vi "CThread Get VI Depends.vi"(4 "Counted Refs":string[](array[string]), 9 "Owning VI":refnum<vi>) -> (3 "Array":refnum<vi>[](array[refnum]))   [LabVIEW 2012, in "CThread.lvlib"]
uses:
  CThread.lvlib
  <vilib>/Utility/traverseref.llb/TRef TravTarget.ctl
  <vilib>/Utility/traverseref.llb/VI Scripting - Traverse.lvlib
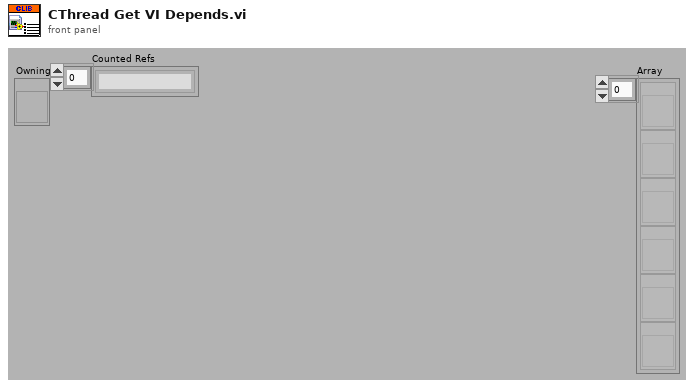
[diagram p1: front panel]
types:
  T1 = typedef "TRef TravTarget.ctl" = enum16{"FP", "BD", "Other"}
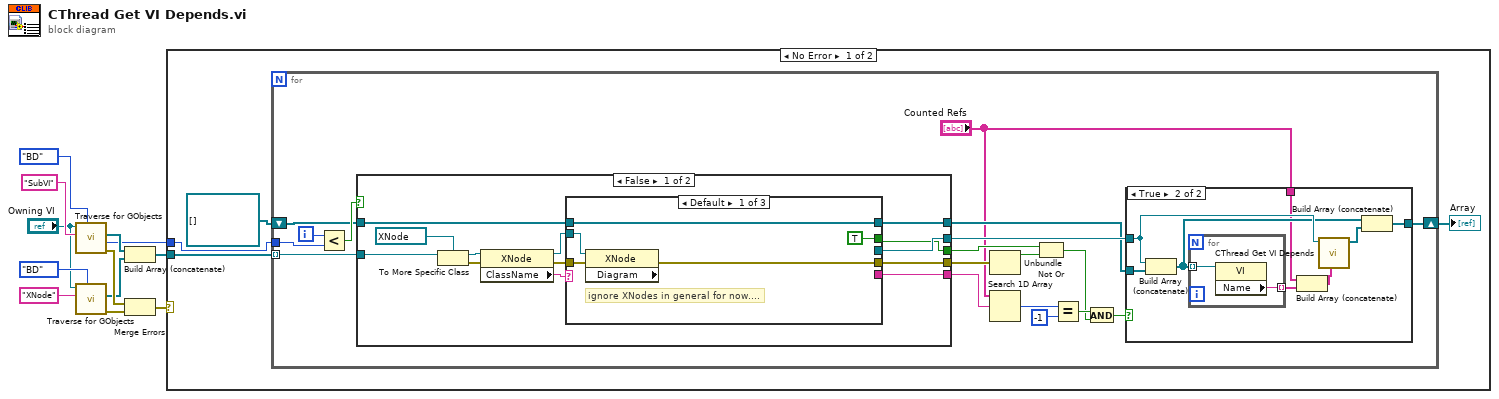
[diagram p0: block diagram]
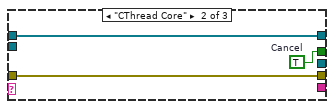
[diagram p2: hidden frame]
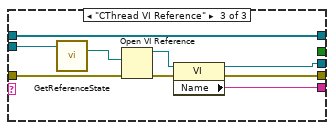
[diagram p3: hidden frame]
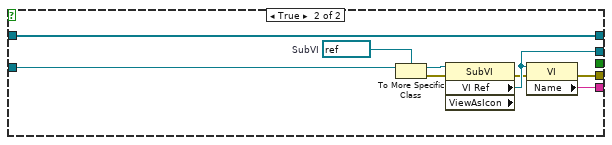
[diagram p4: hidden frame]
diagram:
  n1 = call <vilib>:"Traverse for GObjects.vi"("Traverse Target"=TRef_TravTarget."BD", "Class Name"="SubVI", "VI Refnum"="Owning VI") -> ("error out"=w10:errorcluster, "# of Refs"=w3:i32, "References"=w6:refnum<vi>[])  [unwired: 5 in, 1 out]
  n2 = call <vilib>:"Traverse for GObjects.vi"("Traverse Target"=TRef_TravTarget."BD", "Class Name"="XNode", "VI Refnum"="Owning VI") -> ("error out"=w1:errorcluster, "References"=w5:refnum<vi>[])  [unwired: 5 in, 2 out]
  n3 = Build Array (concatenate)(w6, w5) -> (w4:refnum<vi>[])
  n4 = Merge Errors(w10, w1) -> (w2:errorcluster)
  n5 = case shown="No Error" w2 {
    tunnel: w4 -> [w16 _]
    tunnel: w3 -> [w13 _]
    frame No Error {
      n6 = for {
        tunnel: w16 -> [w34] mode=indexing
        shift-right: [w33] -> w14
        shift-left: refnum<vi>[] [] -> [w27]
        tunnel: w13 -> [w29]
        i -> [w30]
        n7 = Less?(x=w30, y=w29) -> (x < y?=w28:bool)
        n8 = case shown="False" w28 {
          tunnel: w34 -> [w46 w73]
          tunnel: [w41 w70] -> w32
          tunnel: [w40 w69] -> w31
          tunnel: w27 -> [w39 w68]
          tunnel: [w38 w68] -> w26
          tunnel: [w36 _] -> w19
          tunnel: [w35 w67] -> w20
          frame False {
            n9 = To More Specific Class(target class=refnum<vi> refnum ("reference out"), reference=w46) -> (specific class reference=w45:refnum<vi>, error out=w44:errorcluster)  [unwired: 1 in]
            n10 = property class="XNode"(reference=w45, error in=w44) -> (reference out=w42:refnum<vi>, error out=w37:errorcluster, "ClassName"=w43:string)
            n11 = case shown="Default" w43 {
              tunnel: w42 -> [w51 _ w64]
              tunnel: [_ _ w59] -> w41
              tunnel: [_ _ w58] -> w40
              tunnel: w39 -> [w50 w55 w61]
              tunnel: [w50 w55 w61] -> w38
              tunnel: [TRUE ("Cancel") w54 _] -> w36
              tunnel: w37 -> [w52 w53 w60]
              tunnel: [w48 w53 w56] -> w35
              frame Default {
                # "ignore XNodes in general for now...."
                n12 = property class="XNode" props=["Diagram"](reference=w51, error in=w52) -> (error out=w48:errorcluster)  [unwired: 2 out]
              }
              frame "CThread Core" {
                w54 = TRUE  # Cancel
              }
              frame "CThread VI Reference" {
                n13 = call "GetReferenceState.vi"("CThread Reference"=w64) -> ("VI Path"=w63:path)  [unwired: 22 in, 4 out]
                n14 = Open VI Reference(vi path=w63, error in (no error)=w60) -> (vi reference=w62:refnum<vi>, error out=w57:errorcluster)  [unwired: 4 in]
                n15 = property class="VI"(reference=w62, error in=w57) -> (reference out=w59:refnum<vi>, error out=w56:errorcluster, "Name"=w58:string)
              }
            }
          }
          frame True {
            w72 = refnum<vi> refnum  # SubVI
            n16 = To More Specific Class(target class=w72, reference=w73) -> (specific class reference=w71:refnum<vi>, error out=w65:errorcluster)  [unwired: 1 in]
            n17 = property class="SubVI" props=["VI Ref", "ViewAsIcon"](reference=w71, error in=w65) -> (error out=w66:errorcluster, "VI Ref"=w70:refnum<vi>)  [unwired: 2 out]
            n18 = property class="VI"(reference=w70, error in=w66) -> (error out=w67:errorcluster, "Name"=w69:string)  [unwired: 1 out]
          }
        }
        n19 = Unbundle(w20) -> ("status"=w21:bool)  [unwired: 2 out]
        n20 = Search 1D Array(1D array="Counted Refs", element=w31) -> (index of element=w24:i32)  [unwired: 1 in]
        n21 = Not Or(1:w21, 2:w19) -> (0:w18:bool)
        n22 = Equal?(x=w24, y=-1) -> (x = y?=w25:bool)
        n23 = And(x=w25, y=w18) -> (x .and. y?=w22:bool)
        n24 = case shown="True" w22 {
          tunnel: w26 -> [w74 w79]
          tunnel: [w74 w81] -> w33
          tunnel: w32 -> [_ w82]
          tunnel: "Counted Refs" -> [_ w76]
          frame False {
            # "exists or canceled\ndon't add"
          }
          frame True {
            n25 = Build Array (concatenate)(w82, w79) -> (w78:refnum<vi>[])
            n26 = for {
              tunnel: w78 -> [w84] mode=indexing
              tunnel: [w83] -> w77 mode=indexing
              n27 = property class="VI"(reference=w84) -> ("Name"=w83:string)  [unwired: 1 in, 2 out]
            }
            n28 = Build Array (concatenate)(w76, w77) -> (w75:string[])
            n29 = call "CThread Get VI Depends.vi"("Counted Refs"=w75, "Owning VI"=w82) -> ("Array"=w80:refnum<vi>[])  [unwired: 7 in]
            n30 = Build Array (concatenate)(w78, w80) -> (w81:refnum<vi>[])
          }
        }
      }
      "Array" <- w14
    }
    frame Error {
    }
  }
